vi "lvssh2_userauth_publickey_sign_function_handler_64.vi"(9 "lvssh2_userauth_publickey_sign_function":refnum<vi>, 10 "Stop Event Ref":refnum<user-event>, 11 "User Event Ref":refnum<user-event>) -> ()   [LabVIEW 2017, in "libssh2.lvlib"]
uses:
  libssh2.lvlib
  lvssh2_userauth_publickey_sign_function_input_args_64.ctl
  lvssh2_extensions_64.dll
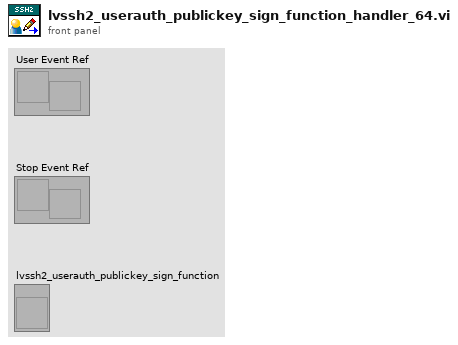
[diagram p1: front panel]
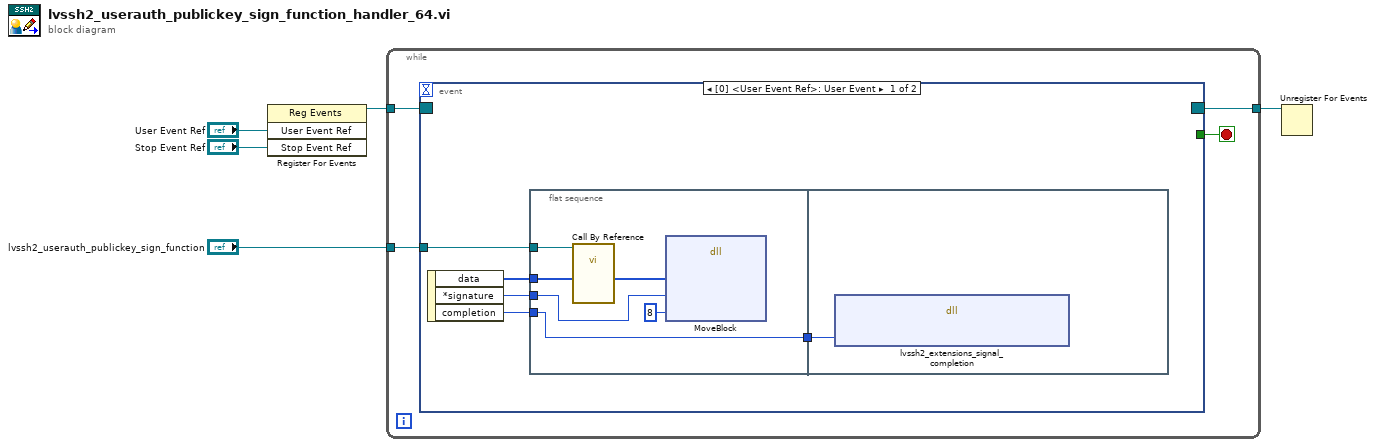
[diagram p0: block diagram]
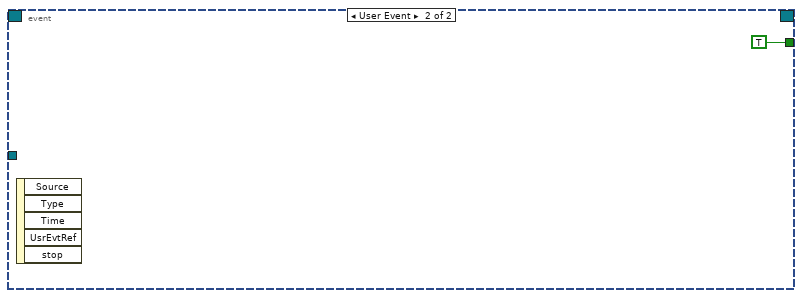
[diagram p2: hidden frame]
diagram:
  n1 = register-events("User Event Ref", "Stop Event Ref") -> (reference out=w4:refnum<event-registration>)  [unwired: 2 in, 1 out]
  n2 = while {
    tunnel: "lvssh2_userauth_publickey_sign_function" -> [w9]
    tunnel: w4 -> [w8]
    tunnel: [w7] -> w1
    stop <- w6 stop-if-true
    n3 = event shown="[0] <User Event Ref>: User Event" {
      selector: w8 -> [_ _]
      dyn-events: [_ _] -> w7
      timeout: _ -> [_ _]
      tunnel: w9 -> [w13 _]
      tunnel: [_ TRUE] -> w6
      event User Event {
        n4 = event-data() -> ("data"=w12:u8[], "*signature"=w11:u64, "completion"=w10:u64)  [unwired: 1 in]
        n5 = flat-sequence {
          tunnel: w13 -> [w20]
          tunnel: w12 -> [w19]
          tunnel: w11 -> [w16]
          tunnel: [w15] -> w14
          tunnel: w10 -> [w15]
          tunnel: w14 -> [w21]
          frame #0 {
            n6 = call-by-ref "?"(reference=w20, "data"=w19) -> ("signature"=w18:u8[])  [unwired: 10 in, 3 out]
            n7 = dll-call lib="LabVIEW" fn="MoveBlock"("ps"=w18, "pd"=w16, "size"=u64 8) -> ()  [unwired: 7 in, 2 out]
          }
          frame #1 {
            n8 = dll-call lib="C:/Users/Pascal/Projects/Home/lvssh2/libssh2/lvssh2_extensions**.*" fn="lvssh2_extensions_signal_completion"("completion"=w21) -> ()  [unwired: 5 in, 2 out]
          }
        }
      }
      event User Event {
        n9 = event-data() -> ()  [unwired: 1 in, 5 out]
      }
    }
  }
  n10 = Unregister For Events(event registration refnum=w1) -> ()  [unwired: 1 in, 1 out]
